vi "Circle fit.vi"() -> ()   [LabVIEW 2023]
doc: "This demonstrates how to use nonlinear curve fitting to fit a circle. This problem is modelled as a 2D curve fit (2 domains, 1 range), where the X and Y data are the noisy points, and Z is 1."
uses:
  <vilib>/gmath/NI_Gmath.lvlib
  <vilib>/Analysis/NI_AALBase.lvlib
panel:
  out "fit y-offset":dbl=0.2
  out "fit x-offset":dbl=0.1
  out "fit radius":dbl=0.3
  out "XY Graph":cluster{"X":dbl[], "Y":dbl[]}[](graph)
  in  "noise sigma":dbl=0.021 format="%.4f"
  in  "radius":dbl=0.3
  in  "y-offset":dbl=0.2
  in  "x-offset":dbl=0.1
  # "Overview: Demonstrates how to fit a circle with the Fitting on a Sphere VI.\nRequirements: LabVIEW Full Development System\nInstructions:\n1. Run the VI.\n2. Change some of the circle parameters and run the VI again."
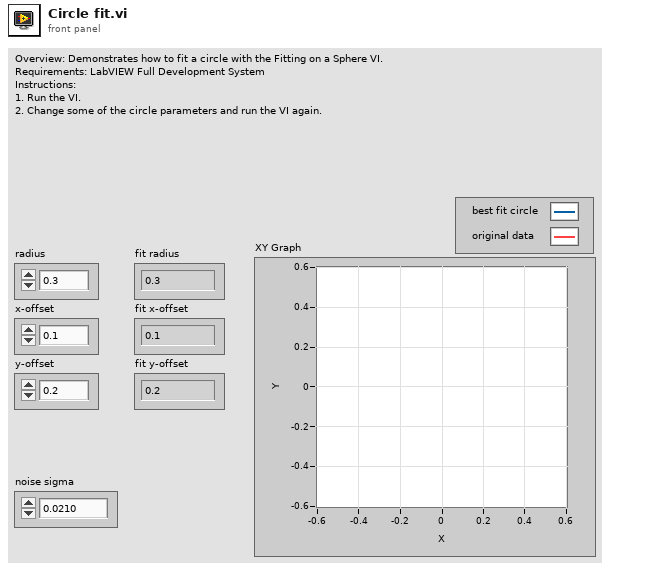
[diagram p1: front panel]
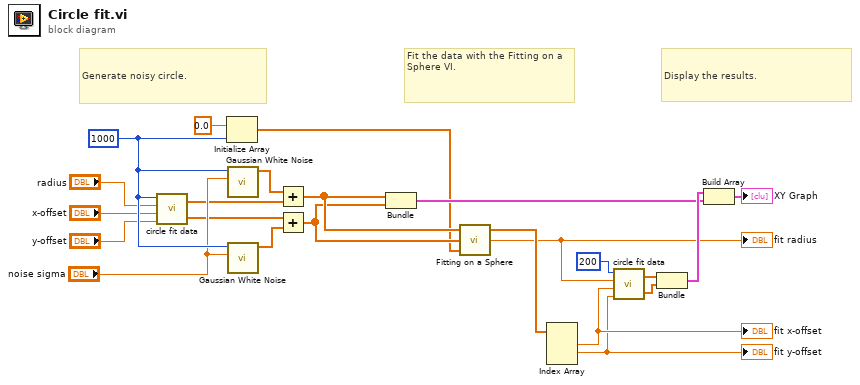
[diagram p0: block diagram]
diagram:
  w23 = 1000 ("samples")
  # "Display the results."
  # "Fit the data with the Fitting on a Sphere VI."
  # "Generate noisy circle."
  n1 = call "circle fit data.vi"("y-offset (b)"="y-offset", "x-offset (a)"="x-offset", "radius"="radius", "samples"=w23) -> ("Y"=w15:dbl[], "X"=w14:dbl[])
  n2 = Initialize Array(0.0, w23) -> (w5:dbl[])
  n3 = call <vilib>:"Gaussian White Noise.vi"("standard deviation"="noise sigma", "samples"=w23) -> ("Gaussian noise pattern"=w20:dbl[])  [unwired: 8 in, 1 out]
  n4 = call <vilib>:"Gaussian White Noise.vi"("standard deviation"="noise sigma", "samples"=w23) -> ("Gaussian noise pattern"=w19:dbl[])  [unwired: 8 in, 1 out]
  n5 = Add(x=w20, y=w14) -> (x+y=w7:dbl[])
  n6 = Add(x=w15, y=w19) -> (x+y=w6:dbl[])
  n7 = Bundle(w7, w6) -> (w8:cluster{dbl[], dbl[]})  [unwired: 1 in]
  n8 = call <vilib>:"Fitting on a Sphere.vi"("Z"=w5, "Y"=w6, "X"=w7) -> ("r"=w3:dbl, "x0, y0, z0"=w4:dbl[])  [unwired: 1 out]
  "fit radius" <- w3
  n9 = Index Array(array=w4) -> (element #1=w2:dbl, element #2=w1:dbl)  [unwired: 3 in, 1 out]
  "fit x-offset" <- w2
  "fit y-offset" <- w1
  n10 = call "circle fit data.vi"("y-offset (b)"=w1, "x-offset (a)"=w2, "radius"=w3, "samples"=200) -> ("Y"=w11:dbl[], "X"=w12:dbl[])
  n11 = Bundle("X"=w12, "Y"=w11) -> (w9:cluster{"X":dbl[], "Y":dbl[]})  [unwired: 1 in]
  n12 = Build Array(w9, w8) -> (→"XY Graph":cluster{"X":dbl[], "Y":dbl[]}[])
